vi "CRYGet Weighting Value.vi"(11 "Weighting Name":string) -> (3 "Weighting Curve":T1={"Name"="", "Curve"=[], "X data"=1, "Y data"=1, "Z data"=1, "X axis"=0, "Y axis"=1, "Z axis"=1, "X unit"="Hz", "Y unit"="", "Z unit"="deg.", "X dB ref"=1.0, "Y dB ref"=1.0, "Z dB ref"=1.0, "single val"=FALSE, "protected"=FALSE, "display X"=TRUE, "display Y"=TRUE, "display Z"=TRUE, "Test Info"="", "Step No."=0, "Plot Settings"={"Color"=0, "Interpolation"=0, "Point Style"=0, "Line Style"=0, "Point Color"=0, "Line Width"=0, "Bar Plot Style"=0, "Fill To"=0}, "AutoProtect"=FALSE} {"Z data" items=["dB", "Lin"]; "X data" items=["dB", "Lin"]; "Y data" items=["dB", "Lin"]; "Z dB ref" format="%.1f"; "Z axis" items=["Log", "Lin"]; "X dB ref" format="%.1f"; "X axis" items=["Log", "Lin"]; "Y axis" items=["Log", "Lin"]; "Y dB ref" format="%.1f"; "Curve"."z" format="%.2f"; "Curve"."y" format="%.2f"; "Curve"."x" format="%.2f"})   [LabVIEW 2013]
uses:
  Typedef Control/CRYData Cluster.ctl
panel:
  in  "Freq, A, B, C wgt.":dbl[][](array[numeric])=[[8.0, 10.0, 12.5, 16.0, 20.0, 25.0, 31.5, 40.0, 50.0, 63.0, 80.0, 100.0, 125.0, 160.0, 200.0, 250.0, 315.0, 400.0, 500.0, 630.0, 800.0, 1000.0, 1250.0, 1600.0, 2000.0, 2500.0, 3150.0, 4000.0, 5000.0, 6300.0, 8000.0, 10000.0, 12500.0, 16000.0, 20000.0, 25000.0, 31500.0, 40000.0, 50000.0, 63000.0, 80000.0, 100000.0], [-77.55000305175781, -70.43000030517578, -63.58000183105469, -56.41999816894531, -50.38999938964844, -44.81999969482422, -39.529998779296875, -34.540000915527344, -30.270000457763672, -26.219999313354492, -22.399999618530273, -19.139999389648438, -16.190000534057617, -13.239999771118164, -10.850000381469727, -8.670000076293945, -6.639999866485596, -4.769999980926514, -3.25, -1.909999966621399, -0.7900000214576721, 0.0, 0.5799999833106995, 0.9900000095367432, 1.2000000476837158, 1.2699999809265137, 1.2000000476837158, 0.9599999785423279, 0.550000011920929, -0.11999999731779099, -1.149999976158142, -2.490000009536743, -4.25, -6.710000038146973, -9.350000381469727, -12.329999923706055, -15.699999809265137, -19.40999984741211, -23.020000457763672, -26.850000381469727, -30.8799991607666, -34.68000030517578], [-43.43000030517578, -38.2400016784668, -33.31999969482422, -28.280000686645508, -24.15999984741211, -20.479999542236328, -17.1299991607666, -14.100000381469727, -11.630000114440918, -9.359999656677246, -7.309999942779541, -5.650000095367432, -4.230000019073486, -2.940000057220459, -2.0399999618530273, -1.3600000143051147, -0.8500000238418579, -0.5, -0.2800000011920929, -0.12999999523162842, -0.03999999910593033, 0.0, 0.009999999776482582, -0.019999999552965164, -0.09000000357627869, -0.20999999344348907, -0.4000000059604645, -0.7300000190734863, -1.1799999475479126, -1.8899999856948853, -2.940000057220459, -4.300000190734863, -6.070000171661377, -8.529999732971191, -11.170000076293945, -14.15999984741211, -17.530000686645508, -21.239999771118164, -24.850000381469727, -28.68000030517578, -32.709999084472656, -36.5099983215332], [-17.59000015258789, -14.329999923706055, -11.34000015258789, -8.430000305175781, -6.21999979019165, -4.440000057220459, -3.0299999713897705, -1.9800000190734863, -1.2999999523162842, -0.8199999928474426, -0.5, -0.30000001192092896, -0.17000000178813934, -0.07999999821186066, -0.029999999329447746, 0.0, 0.019999999552965164, 0.029999999329447746, 0.029999999329447746, 0.029999999329447746, 0.019999999552965164, 0.0, -0.029999999329447746, -0.09000000357627869, -0.17000000178813934, -0.30000001192092896, -0.5, -0.8299999833106995, -1.2899999618530273, -1.9900000095367432, -3.049999952316284, -4.409999847412109, -6.179999828338623, -8.630000114440918, -11.279999732971191, -14.260000228881836, -17.639999389648438, -21.350000381469727, -24.950000762939453, -28.790000915527344, -32.81999969482422, -36.619998931884766]] format="%.2f"
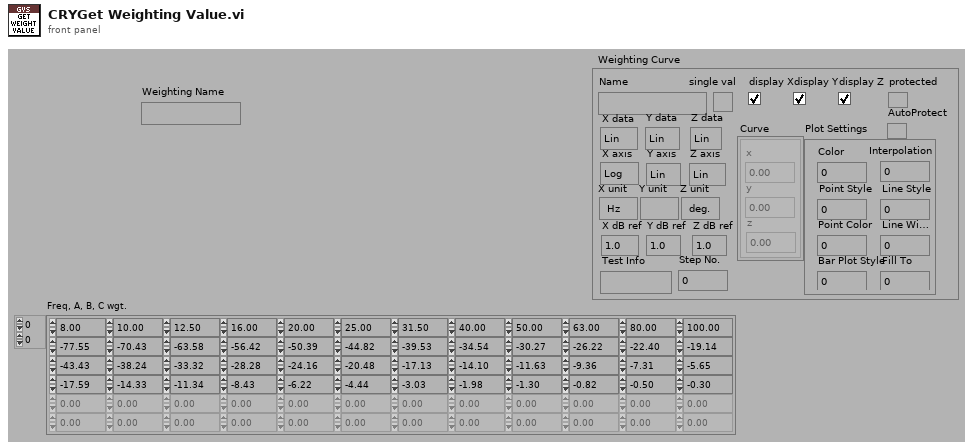
[diagram p1: front panel]
types:
  T1 = typedef "CRYData Cluster.ctl" = cluster{"Name":string, "Curve":cluster{"x":dbl, "y":dbl, "z":dbl}[], "X data":u16, "Y data":u16, "Z data":u16, "X axis":u16, "Y axis":u16, "Z axis":u16, "X unit":string, "Y unit":string, "Z unit":string, "X dB ref":dbl, "Y dB ref":dbl, "Z dB ref":dbl, "single val":bool, "protected":bool, "display X":bool, "display Y":bool, "display Z":bool, "Test Info":string, "Step No.":i32, "Plot Settings":cluster{"Color":u32, "Interpolation":u8, "Point Style":u8, "Line Style":u8, "Point Color":u32, "Line Width":u8, "Bar Plot Style":u8, "Fill To":i16}, "AutoProtect":bool}
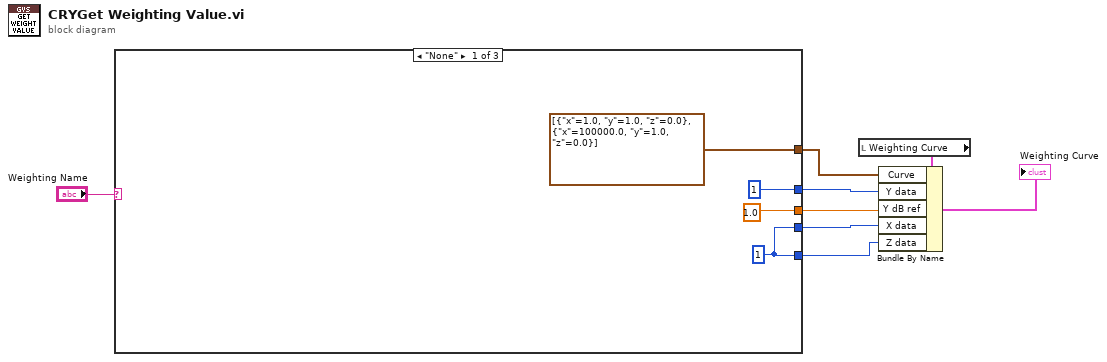
[diagram p0: block diagram]
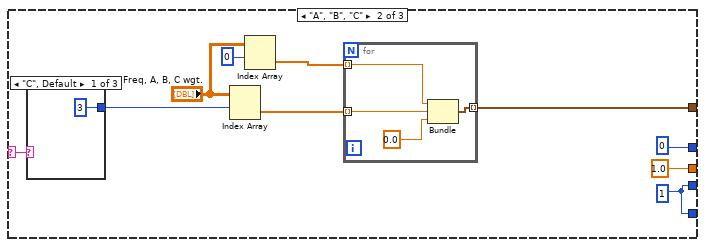
[diagram p2: hidden frame]
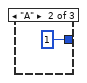
[diagram p3: hidden frame]
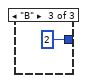
[diagram p4: hidden frame]
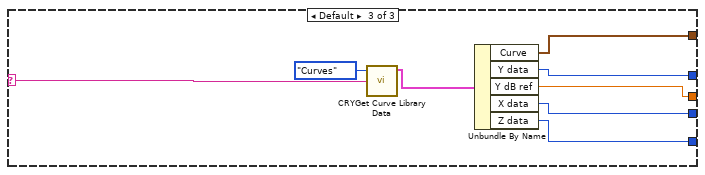
[diagram p5: hidden frame]
diagram:
  n1 = case shown="\"None\"" "Weighting Name" {
    selector: "Weighting Name" -> [_ w18 w35]
    tunnel: [cluster{"x":dbl, "y":dbl, "z":dbl}[] [{"x"=1.0, "y"=1.0, "z"=0.0}, {"x"=100000.0, "y"=1.0, "z"=0.0}] ("Weight") w16 w34] -> w7
    tunnel: [1.0 ("Y dB ref") 1.0 ("Y dB ref") w32] -> w4
    tunnel: [u16 1 ("Y data") u16 0 ("Y data") w33] -> w3
    tunnel: [w9 w13 w31] -> w2
    tunnel: [w9 w13 w30] -> w1
    frame "None" {
      w9 = u16 1 ("X data")
    }
    frame "A", "B", "C" {
      w13 = u16 1 ("X data")
      n2 = case shown="\"C\", Default" w18 {
        tunnel: [3 ("index (row)") 1 ("index (row)") 2 ("index (row)")] -> w17
        frame "C", Default {
        }
        frame "A" {
        }
        frame "B" {
        }
      }
      n3 = Index Array(array="Freq, A, B, C wgt.", index (row)=w17) -> (element=w22:dbl[])  [unwired: 1 in]
      n4 = Index Array(array="Freq, A, B, C wgt.", index (row)=0) -> (element=w21:dbl[])  [unwired: 1 in]
      n5 = for {
        tunnel: w21 -> [w29] mode=indexing
        tunnel: w22 -> [w26] mode=indexing
        tunnel: [w28] -> w16 mode=indexing
        n6 = Bundle(w29, w26, "Lin Out"=0.0) -> (w28:cluster{dbl, dbl, "Lin Out":dbl})  [unwired: 1 in]
      }
    }
    frame Default {
      n7 = call "CRYGet Curve Library Data.vi"("Type"=enum16{"Curves", "Values", "Results", "WFM"}."Curves", "Data Name"=w35) -> ("Curve"=w36:T1)  [unwired: 4 out]
      n8 = Unbundle By Name(w36) -> ("Curve"=w34:cluster{"x":dbl, "y":dbl, "z":dbl}[], "Y data"=w33:u16, "Y dB ref"=w32:dbl, "X data"=w31:u16, "Z data"=w30:u16)
    }
  }
  n9 = local read "Weighting Curve"() -> (w6:T1)
  n10 = Bundle By Name(cluster=w6, "Curve"=w7, "Y data"=w3, "Y dB ref"=w4, "X data"=w2, "Z data"=w1) -> (→"Weighting Curve":T1)
